vi "Write Current Parameter.vi"(8 "error in (no error)":errorcluster, 10 "AbstractData.lvclass":refnum<class "AbstractData.lvclass">, 11 "AbstractExtractor in":refnum<class "AbstractExtractor.lvclass">) -> (0 "error out":errorcluster, 3 "AbstractExtractor out":refnum<class "AbstractExtractor.lvclass">)   [LabVIEW 2014, in "AbstractExtractor.lvclass"]
uses:
  AbstractExtractor.lvclass
  Model/Data/AbstractData/AbstractData.lvclass
  AbstractExtractor.lvclass/AbstractExtractor.ctl
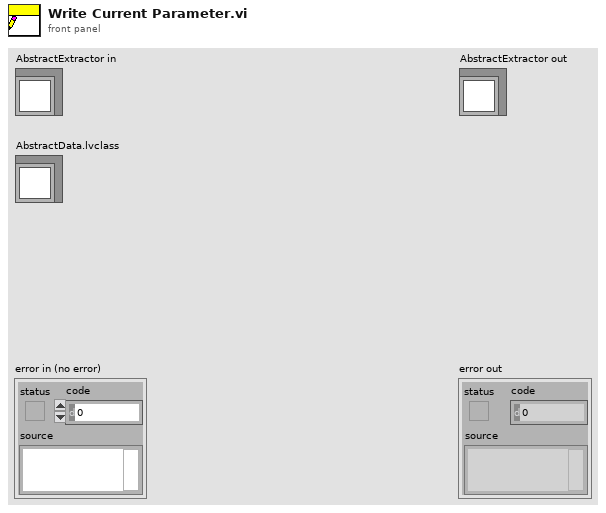
[diagram p1: front panel]
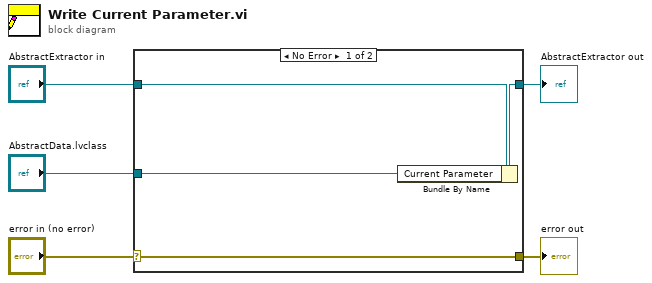
[diagram p0: block diagram]
diagram:
  n1 = case shown="No Error" "error in (no error)" {
    selector: "error in (no error)" -> [w9 w10]
    tunnel: [w9 w10] -> w4
    tunnel: [w7 w11] -> w2
    tunnel: "AbstractExtractor in" -> [w8 w11]
    tunnel: "AbstractData.lvclass" -> [w6 _]
    frame No Error {
      n2 = Bundle By Name(cluster=w8, "Current Parameter"=w6) -> (w7:refnum<class "AbstractExtractor.lvclass">)
    }
    frame Error {
    }
  }
  "error out" <- w4
  "AbstractExtractor out" <- w2
